vi "list box selected cell.vi"(10 "Coords":T2, 11 "MulticolumnListbox in":refnum<vi>) -> (0 "error out":errorcluster, 1 "cell position":T1, 2 "value":string, 3 "tag select name":string)   [LabVIEW 2013, in "tag select module editor node.lvclass"]
uses:
  tag select module editor node.lvclass
  <vilib>/Utility/miscctls.llb/LVPoint32TypeDef.ctl
  <vilib>/Utility/miscctls.llb/LVRowAndColumnTypeDef.ctl
  Table API/Source/Listbox/Multi Column Listbox.lvclass
panel:
  in  "error in":errorcluster
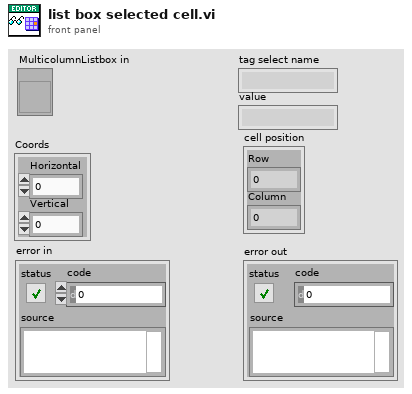
[diagram p1: front panel]
types:
  T1 = typedef "LVRowAndColumnTypeDef.ctl" = cluster{"Row":i32, "Column":i32}
  T2 = typedef "LVPoint32TypeDef.ctl" = cluster{"Horizontal":i32, "Vertical":i32}
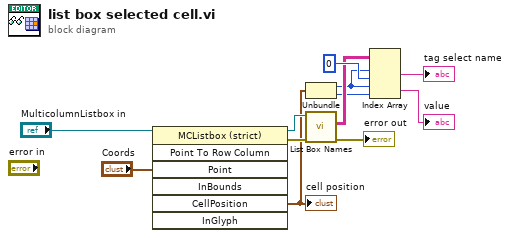
[diagram p0: block diagram]
diagram:
  n1 = invoke class="MCListbox (strict)" method="Point To Row Column"(reference="MulticolumnListbox in", "Point"="Coords") -> (reference out=w6:refnum<vi>, error out=w7:errorcluster, "CellPosition"=w5:T1)  [unwired: 5 in, 4 out]
  "cell position" <- w5
  n2 = Unbundle(w5) -> ("Row"=w4:i32, "Column"=w3:i32)
  n3 = call "List Box Names.vi"("error in (no error)"=w7, "MulticolumnListbox in"=w6) -> ("error out"=→"error out":errorcluster, "ItemNames"=w8:string[][])  [unwired: 7 in, 1 out]
  n4 = Index Array(array=w8, index (row) #1=w4, index (col) #1=0 ("disabled index (col)"), index (row) #2=w4, index (col) #2=w3) -> (element #1=→"tag select name":string, element #2=→"value":string)
